vi "Converter_get_baseline_DBL_arr.vi"(10 "From unit #":i32, 11 "Average array in":dbl[][](array[numeric])) -> (3 "baselines for evaluation":dbl[](array[numeric]))   [LabVIEW 2013]
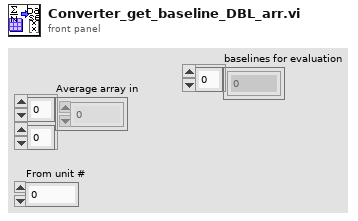
[diagram p1: front panel]
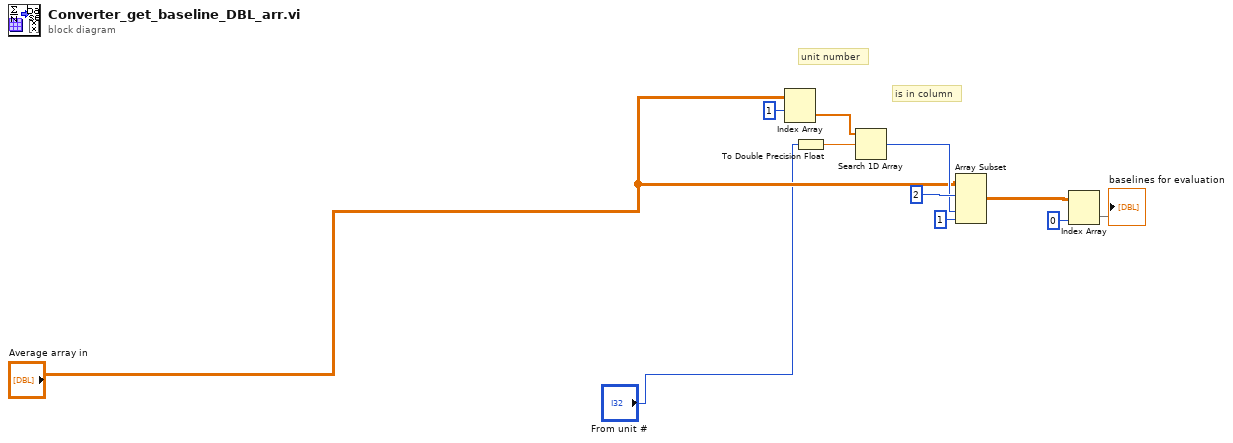
[diagram p0: block diagram]
diagram:
  # "is in column"
  # "unit number"
  n1 = Index Array(array="Average array in", index (row)=1) -> (element=w8:dbl[])  [unwired: 1 in]
  n2 = To Double Precision Float(number="From unit #") -> (double precision float=w6:dbl)
  n3 = Search 1D Array(1D array=w8, element=w6) -> (index of element=w10:i32)  [unwired: 1 in]
  n4 = Array Subset(array="Average array in", index (row)=2 ("index"), index (col)=w10, length (col)=1 ("length")) -> (w3:dbl[][])  [unwired: 1 in]
  n5 = Index Array(array=w3, index (col)=0 ("disabled index (col)")) -> (element=→"baselines for evaluation":dbl[])  [unwired: 1 in]
